vi "_attribute_read.vi"(5 "Repeated Capability":string, 7 "Query Parameter (None)":string, 8 "error in":errorcluster caption="error in (no error)", 10 "Attribute ID":string, 11 "VISA resource name":refnum<visa-resource-name>) -> (0 "error out":errorcluster, 1 "Double out":dbl, 2 "Int32 out":i32, 3 "VISA resource name out":refnum<visa-resource-name>, 4 "Boolean out":bool, 6 "String out":string, 9 "Int64 out":i64)   [LabVIEW 2020, in "Rohde&Schwarz RTx Oscilloscopes.lvlib" / "rsidr_core.lvlib"]
uses:
  rsidr_core.lvlib
  type_Error_Codes.ctl
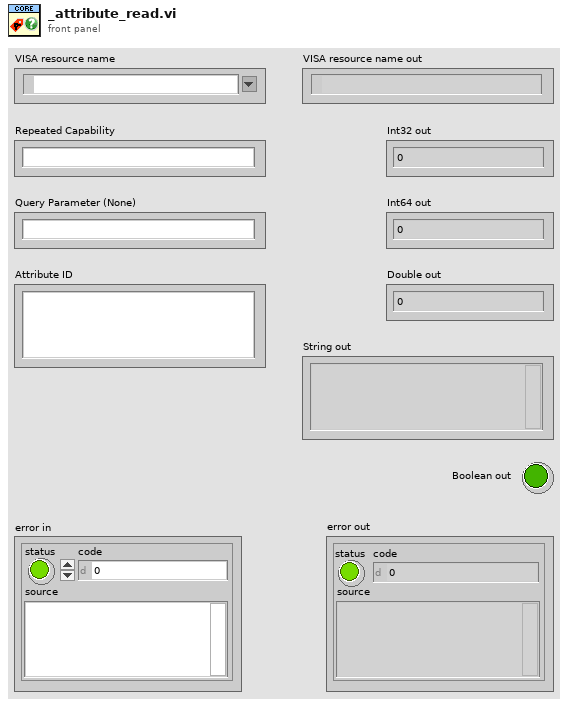
[diagram p1: front panel]
types:
  T1 = typedef "Rohde&Schwarz RTx Oscilloscopes.lvlib/rsidr_core.lvlib/type_Error_Codes.ctl" = enum16{"No_error", "VISA_err_ResourceNotFound", "VISA_err_Timeout", "VISA_warn_MoreDataAvailable", "RS_err_MissingCallback", "RS_err_InvalidAttribute", "RS_err_InvalidValue", "RS_err_UnknownResource", "RS_err_AlreadyInitialized", "RS_err_InstrumentStatus", "RS_err_BadRepCapName", "RS_err_TypesMismatch", "RS_err_ValueNotSupported", "RS_err_InvalidRngTable", "RS_err_IDqueryFail", "RS_err_UnexpResponse", "VISA_warn_ConfigNotLoaded", "RS_err_AttributeNotReadable", "RS_err_AttributeNotWritable", "RS_err_InstrumentType", "RS_err_InstrumentOption", "VISA_err_InvalidSize", "RS_err_ReliabilityIndicator", "VISA_warn_UnknownStatus", "VISA_warn_TermCharRead", "VISA_err_IO_error", "RS_err_FunctionNotSupported", "VISA_warn_QueueEmpty"}
  T2 = typedef "Rohde&Schwarz RTx Oscilloscopes.lvlib/rsidr_core.lvlib/type_Attribute.ctl" = cluster{"Identifier":string, "Descriptive Name":string, "Data Type":T3, "Command":string, "Access":T4, "Range Table":string, "Read Callback":string, "Write Callback":string, "Supported Models":string, "Instrument Options":string, "Index":i32, "OPC Wait":bool, "No Status Check":bool, "Cache Only":bool}
  T3 = typedef "Rohde&Schwarz RTx Oscilloscopes.lvlib/rsidr_core.lvlib/type_Attribute_Data_Type.ctl" = enum16{"Integer 32", "Double", "String", "Boolean", "None", "Integer 64", "RawString"}
  T4 = typedef "Rohde&Schwarz RTx Oscilloscopes.lvlib/rsidr_core.lvlib/type_ReadWriteAccess.ctl" = enum16{"Read Only", "Write Only", "Read/Write"}
  T5 = typedef "Rohde&Schwarz RTx Oscilloscopes.lvlib/rsidr_core.lvlib/type_Session_Data.ctl" = cluster{"IDN string":string, "Instrument FW":string, "Instr type":string, "Instr type for err. msg.":string, "Installed Options":string[], "Ignore Error Messages":string, "Logging params":variant, "OPC Timeout":i32, "VISA Timeout":i32, "STB Poll VISA Timeout":i32, "Additional Flags":i32, "Wait Before Read":i32, "Wait Before Write":i32, "Option String Flags":i32, "IO Segment Size":i64, "VISA Access Mode":T6, "Interface Type":T7, "OPC Wait Mode":T8, "Bin Float Number  Format":T9, "Bin Integer Number Format":T10, "Simulate":bool, "VXIcapable":bool, "Duplicate Session":bool, "Add LF to Write":bool, "Logging":bool, "Fast Sweep":bool, "Query Instrument Status":bool, "Check Range":bool, "Check Options":bool, "OPC-sync Attr Writes":bool, "OPC-sync Attr Queries":bool}
  T6 = typedef "Rohde&Schwarz RTx Oscilloscopes.lvlib/rsidr_core.lvlib/type_VisaAccessMode.ctl" = u16
  T7 = typedef "Rohde&Schwarz RTx Oscilloscopes.lvlib/rsidr_core.lvlib/type_InterfaceType.ctl" = enum16{"Unknown", "GPIB", "VXI", "GPIB_VXI", "ASRL", "PXI", "TCPIP", "USB", "SOCKET"}
  T8 = typedef "Rohde&Schwarz RTx Oscilloscopes.lvlib/rsidr_core.lvlib/type_OPC_Wait_Mode.ctl" = enum16{"STBpolling", "STBpollingSlow", "STBpollingSuperSlow", "ServiceRequest", "OPCquery"}
  T9 = typedef "Rohde&Schwarz RTx Oscilloscopes.lvlib/rsidr_core.lvlib/type_Binary_Float_Number_Format.ctl" = enum16{"Float_4_Bytes_Swapped", "Float_4_Bytes", "Double_8_Bytes_Swapped", "Double_8_Bytes"}
  T10 = typedef "Rohde&Schwarz RTx Oscilloscopes.lvlib/rsidr_core.lvlib/type_Binary_Integer_Number_Format.ctl" = enum16{"Int32_4_Bytes_Swapped", "Int32_4 Bytes", "Int16_2_Bytes_Swapped", "Int16_2_Bytes"}
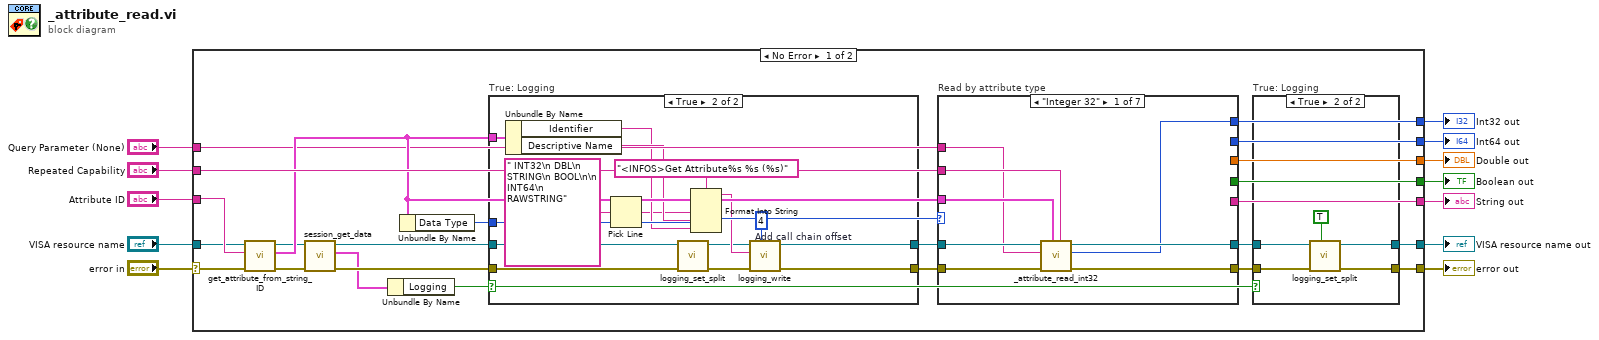
[diagram p0: block diagram]
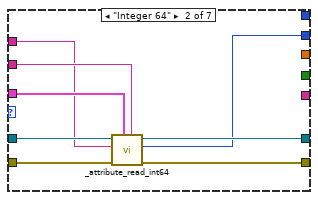
[diagram p4: hidden frame]
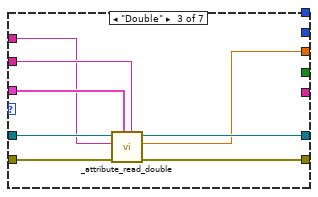
[diagram p5: hidden frame]
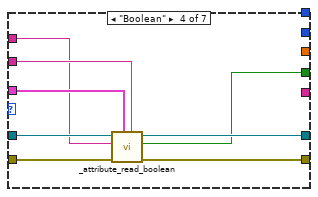
[diagram p6: hidden frame]
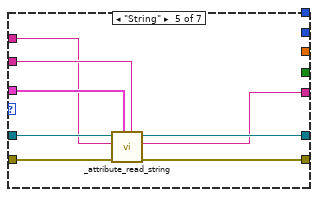
[diagram p7: hidden frame]
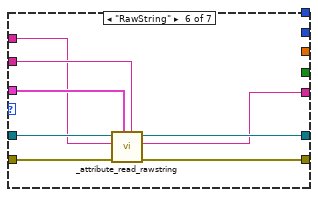
[diagram p8: hidden frame]
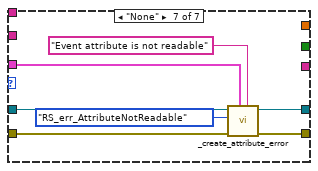
[diagram p9: hidden frame]
diagram:
  n1 = case shown="No Error" "error in" {
    selector: "error in" -> [w19 w116]
    tunnel: "VISA resource name" -> [w15 w117]
    tunnel: "Repeated Capability" -> [w36 _]
    tunnel: [w26 w117] -> w10
    tunnel: [w27 w116] -> w9
    tunnel: "Attribute ID" -> [w17 _]
    tunnel: [w35 _] -> w6
    tunnel: [w34 _] -> w5
    tunnel: [w33 _] -> w4
    tunnel: [w32 _] -> w3
    tunnel: [w31 _] -> w2
    tunnel: "Query Parameter (None)" -> [w13 _]
    frame No Error {
      n2 = call "get_attribute_from_string_ID.vi"("error in"=w19, "Attribute ID in"=w17, "VISA resource name"=w15) -> ("error out"=w18:errorcluster, "Attribute out"=w16:T2, "VISA resource name out"=w14:refnum<visa-resource-name>)  [unwired: 6 in]
      n3 = call "session_get_data.vi"("error in"=w18, "VISA resource name"=w14) -> ("error out"=w25:errorcluster, "Session User Data out"=w21:T5, "VISA resource name out"=w24:refnum<visa-resource-name>)  [unwired: 6 in, 1 out]
      n4 = Unbundle By Name(w21) -> ("Logging"=w23:bool)
      n5 = Unbundle By Name(w16) -> ("Data Type"=w22:T3)
      n6 = case "True: Logging" shown="True" w23 {
        tunnel: w25 -> [w37 w41]
        tunnel: w16 -> [_ w53]
        tunnel: w24 -> [w38 w42]
        tunnel: [w38 w44] -> w30
        tunnel: w22 -> [_ w48]
        tunnel: [w37 w43] -> w20
        frame False {
        }
        frame True {
          w45 = 4  # Add call chain offset
          n7 = Unbundle By Name(w53) -> ("Identifier"=w50:string, "Descriptive Name"=w51:string)
          n8 = Pick Line(multi-line string=" INT32\n DBL\n STRING\n BOOL\n\n INT64\n RAWSTRING", line index=w48) -> (output string=w47:string)  [unwired: 1 in]
          n9 = call "logging_set_split.vi"("error in"=w41, "VISA resource name"=w42) -> ("error out"=w40:errorcluster, "VISA resource name out"=w39:refnum<visa-resource-name>)  [unwired: 8 in]
          n10 = Format Into String(format string="<INFOS>Get Attribute%s %s (%s)", w47, w51, w50) -> (resulting string=w49:string)  [unwired: 2 in, 1 out]
          n11 = call "logging_write.vi"("Add call chain offset\n(No call chain)"=w45, "error in"=w40, "String to write"=w49, "VISA resource name"=w39) -> ("error out"=w43:errorcluster, "VISA resource name out"=w44:refnum<visa-resource-name>)  [unwired: 6 in]
        }
      }
      n12 = case "Read by attribute type" shown="\"Integer 32\"" w22 {
        tunnel: w16 -> [w62 w71 w78 w87 w95 w103 w113]
        tunnel: w30 -> [w68 w76 w84 w92 w100 w108 w112]
        tunnel: w20 -> [w67 w75 w83 w91 w99 w107 w115]
        tunnel: w36 -> [w63 w72 w79 w88 w96 w104 _]
        tunnel: [w66 w74 w82 w90 w98 w106 w111] -> w28
        tunnel: [w65 w73 w81 w89 w97 w105 w114] -> w29
        tunnel: [w64 _ _ _ _ _ _] -> w35
        tunnel: [_ w70 _ _ _ _ _] -> w34
        tunnel: [_ _ w80 _ _ _ _] -> w33
        tunnel: [_ _ _ w86 _ _ _] -> w32
        tunnel: [_ _ _ _ w94 w102 _] -> w31
        tunnel: w13 -> [w61 w69 w77 w85 w93 w101 _]
        frame "Integer 32" {
          n13 = call "_attribute_read_int32.vi"("Repeated Capability"=w63, "Attribute"=w62, "error in"=w67, "Query Parameter"=w61, "VISA resource name"=w68) -> ("error out"=w65:errorcluster, "Int32 out"=w64:i32, "VISA resource name out"=w66:refnum<visa-resource-name>)  [unwired: 4 in]
        }
        frame "Integer 64" {
          n14 = call "_attribute_read_int64.vi"("Repeated Capability"=w72, "Attribute"=w71, "error in"=w75, "Query Parameter"=w69, "VISA resource name"=w76) -> ("error out"=w73:errorcluster, "Int64 out"=w70:i64, "VISA resource name out"=w74:refnum<visa-resource-name>)  [unwired: 4 in]
        }
        frame "Double" {
          n15 = call "_attribute_read_double.vi"("Repeated Capability"=w79, "Attribute"=w78, "error in"=w83, "Query Parameter"=w77, "VISA resource name"=w84) -> ("error out"=w81:errorcluster, "Double out"=w80:dbl, "VISA resource name out"=w82:refnum<visa-resource-name>)  [unwired: 4 in]
        }
        frame "Boolean" {
          n16 = call "_attribute_read_boolean.vi"("Repeated Capability"=w88, "Attribute"=w87, "error in"=w91, "Query Parameter"=w85, "VISA resource name"=w92) -> ("error out"=w89:errorcluster, "Boolean out"=w86:bool, "VISA resource name out"=w90:refnum<visa-resource-name>)  [unwired: 4 in]
        }
        frame "String" {
          n17 = call "_attribute_read_string.vi"("Repeated Capability"=w96, "Attribute"=w95, "error in"=w99, "Query Parameter"=w93, "VISA resource name"=w100) -> ("error out"=w97:errorcluster, "String out"=w94:string, "VISA resource name out"=w98:refnum<visa-resource-name>)  [unwired: 4 in]
        }
        frame "RawString" {
          n18 = call "_attribute_read_rawstring.vi"("Repeated Capability"=w104, "Attribute"=w103, "error in"=w107, "Query Parameter"=w101, "VISA resource name"=w108) -> ("error out"=w105:errorcluster, "String out"=w102:string, "VISA resource name out"=w106:refnum<visa-resource-name>)  [unwired: 4 in]
        }
        frame "None" {
          n19 = call "_create_attribute_error.vi"("Error Elaboration (\"\")"="Event attribute is not readable" ("Error Elaboration"), "Attribute"=w113, "error in"=w115, "Error Enum in"=type_Error_Codes."RS_err_AttributeNotReadable" ("Error Enum in (from err to recompose)"), "VISA resource name"=w112) -> ("error out"=w114:errorcluster, "VISA resource name out"=w111:refnum<visa-resource-name>)  [unwired: 5 in]
        }
      }
      n20 = case "True: Logging" shown="True" w23 {
        tunnel: w29 -> [w55 w60]
        tunnel: [w55 w58] -> w27
        tunnel: w28 -> [w54 w59]
        tunnel: [w54 w57] -> w26
        frame False {
        }
        frame True {
          n21 = call "logging_set_split.vi"("Evaluate section error (F)"=TRUE, "error in"=w60, "VISA resource name"=w59) -> ("error out"=w58:errorcluster, "VISA resource name out"=w57:refnum<visa-resource-name>)  [unwired: 7 in]
        }
      }
    }
    frame Error {
    }
  }
  "error out" <- w9
  "VISA resource name out" <- w10
  "Int64 out" <- w5
  "Int32 out" <- w6
  "Double out" <- w4
  "String out" <- w2
  "Boolean out" <- w3
